vi "Speech-WpnAltSpd-Talk.vi"(1 "Ground Speed":i32, 2 "Altitude":i32, 3 "Current WP":i32) -> (0 "Text":string)   [LabVIEW 8.6]
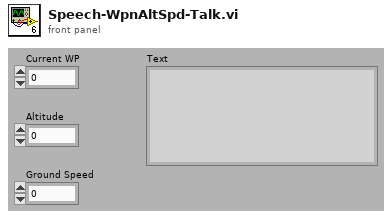
[diagram p1: front panel]
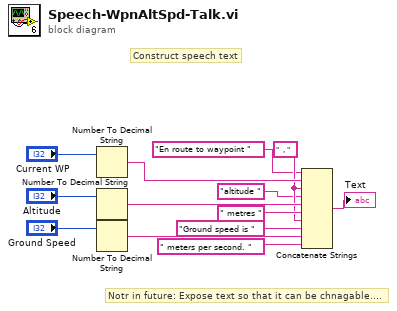
[diagram p0: block diagram]
diagram:
  w5 = "  , " ("string")
  # "Notr in future: Expose text so that it can be chnagable...."
  # "Construct speech text"
  n1 = Number To Decimal String(number="Current WP") -> (decimal integer string=w9:string)  [unwired: 1 in]
  n2 = Number To Decimal String(number="Altitude") -> (decimal integer string=w10:string)  [unwired: 1 in]
  n3 = Number To Decimal String(number="Ground Speed") -> (decimal integer string=w12:string)  [unwired: 1 in]
  n4 = Concatenate Strings("En route to waypoint " ("F-format string 3"), w9, w5, "altitude " ("string"), w10, " metres " ("F-format string 3"), w5, "Ground speed is " ("string"), w12, " meters per second. " ("F-format string 3")) -> (→"Text":string)
